vi "Constant Array Size Sha-1.vi"(11 "Message In as Byte Array":u8[](array[numeric])=[97, 0, 0, 0, 0, 0, 0, 0, 0, 0, 0, 0, 0, 0, 0, 0, 0, 0, 0, 0, 0, 0, 0, 0, 0, 0, 0, 0, 0, 0, 0, 0, 0, 0, 0, 0, 0, 0, 0, 0, 0, 0, 0, 0, 0, 0, 0, 0, 0, 0, 0, 0, 0, 0, 0, 0, 0, 0, 0, 0, 0, 0, 0, 0, 0]) -> (3 "Digest":u8[](array[numeric]) format="%x")   [LabVIEW 2014]
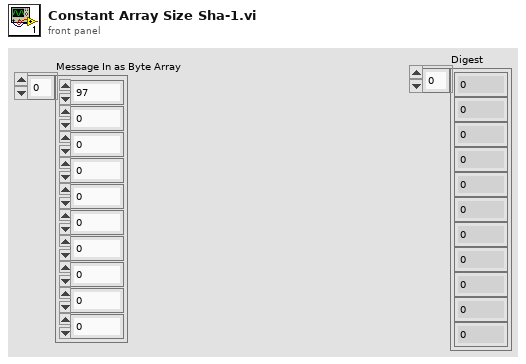
[diagram p1: front panel]
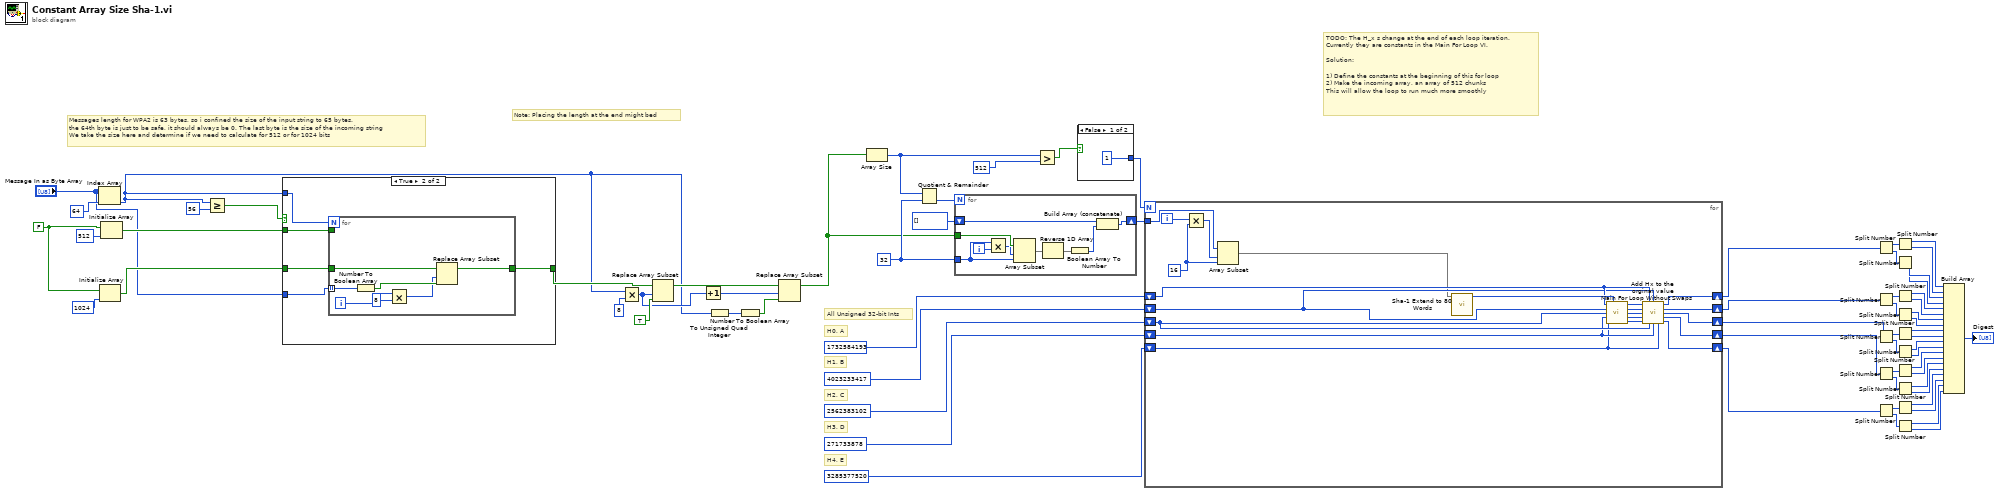
[diagram p0: block diagram]
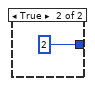
[diagram p2: hidden frame]
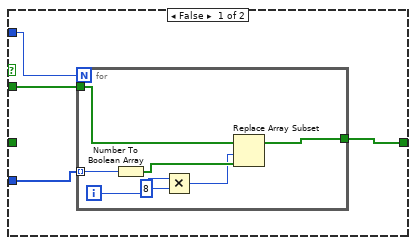
[diagram p3: hidden frame]
diagram:
  w8 = 32 ("y")
  w66 = FALSE
  # "Note: Placing the length at the end might bed"
  # "All Unsigned 32-bit Ints"
  # "H0, A"
  # "H3, D"
  # "H4, E"
  # "H2, C"
  # "H1, B"
  # "TODO: The H_x s change at the end of each loop iteration. \nCurrently they are constants in the Main For Loop VI. \n\nSolution:\n\n1) Define the constants at the beginning of this for loop\n2) Make the incoming array, an array of 512 chunks\nThis will allow the loop to run much more smoothly"
  # "Messages length for WPA2 is 63 bytes, so i confined the size of the input string to 65 bytes. \nthe 64th byte is just to be safe, it should always be 0. The last byte is the size of the incoming string\nWe take the size here and determine if we need to calculate for 512 or for 1024 bits"
  n1 = Index Array(array="Message In as Byte Array", index=64) -> (element=w53:u8)
  n2 = Initialize Array(w66, 1024 ("dimension size")) -> (w62:bool[])
  n3 = Initialize Array(w66, 512 ("dimension size")) -> (w61:bool[])
  n4 = Greater Or Equal?(x=w53, y=u8 56) -> (x >= y?=w63:bool)
  n5 = case shown="True" w63 {
    tunnel: w62 -> [_ w80]
    tunnel: w61 -> [w72 w84]
    tunnel: w53 -> [w70 w81]
    tunnel: "Message In as Byte Array" -> [w71 w83]
    tunnel: [w69 w82] -> w59
    frame False {
      n6 = for {
        N: w70 -> [_]
        tunnel: w72 -> [w78]
        tunnel: w71 -> [w79] mode=indexing
        tunnel: [w73] -> w69
        i -> [w76]
        n7 = Number To Boolean Array(number=w79) -> (Boolean array=w77:bool[])
        n8 = Multiply(x=w76, y=8) -> (x*y=w74:i32)
        n9 = Replace Array Subset(array=w78, new element=w77, index=w74) -> (w73:bool[])
      }
    }
    frame True {
      n10 = for {
        N: w81 -> [_]
        tunnel: w84 -> [_]
        tunnel: w83 -> [w91] mode=indexing
        tunnel: [w86] -> w82
        tunnel: w80 -> [w85]
        i -> [w89]
        n11 = Number To Boolean Array(number=w91) -> (Boolean array=w90:bool[])
        n12 = Multiply(x=w89, y=8) -> (x*y=w87:i32)
        n13 = Replace Array Subset(array=w85, new element=w90, index=w87) -> (w86:bool[])
      }
    }
  }
  n14 = Multiply(x=w53, y=8) -> (x*y=w54:i32)
  n15 = Replace Array Subset(array=w59, new element=TRUE, index=w54) -> (w56:bool[])
  n16 = Increment(x=w54) -> (x+1=w55:i32)
  n17 = To Unsigned Quad Integer(1:w53) -> (0:w52:u64)
  n18 = Number To Boolean Array(number=w52) -> (Boolean array=w51:bool[])
  n19 = Replace Array Subset(array=w56, new element=w51, index=w55) -> (w5:bool[])
  n20 = Array Size(array=w5) -> (size(s)=w3:i32)
  n21 = Quotient & Remainder(x=w3, y=w8) -> (floor(x/y)=w9:i32)  [unwired: 1 out]
  n22 = for {
    N: w9 -> [_]
    tunnel: w5 -> [w100]
    tunnel: w8 -> [w96]
    shift-right: [w94] -> w6
    shift-left: u32[] [] -> [w93]
    i -> [w98]
    n23 = Multiply(x=w96, y=w98) -> (x*y=w97:i32)
    n24 = Array Subset(array=w100, index=w97, length=w96) -> (w99:bool[])
    n25 = Reverse 1D Array(array=w99) -> (reversed array=w95:bool[])
    n26 = Boolean Array To Number(Boolean array=w95) -> (number=w92:u32)
    n27 = Build Array (concatenate)(w93, w92) -> (w94:u32[])
  }
  n28 = Greater?(x=w3, y=512) -> (0:w2:bool)
  n29 = case shown="False" w2 {
    tunnel: [1 2] -> w1
    frame False {
    }
    frame True {
    }
  }
  n30 = for {
    N: w1 -> [_]
    shift-right: [w118] -> w45
    shift-left: u32 1732584193 -> [w112]
    shift-right: [w117] -> w32
    shift-left: u32 4023233417 -> [w111]
    shift-right: [w116] -> w23
    shift-left: u32 2562383102 -> [w110]
    shift-right: [w115] -> w22
    shift-left: u32 271733878 -> [w109]
    shift-right: [w114] -> w19
    shift-left: u32 3285377520 -> [w108]
    tunnel: w6 -> [w104]
    i -> [w107]
    w106 = 16 ("length")
    n31 = Multiply(x=w107, y=w106) -> (x*y=w105:i32)
    n32 = Array Subset(array=w104, index=w105, length=w106) -> (w103:u32[])
    n33 = call "Sha-1 Extend to 80 Words.vi"("16 32-bit Words In"=w103) -> ("80 32 Bit Words Out"=w113:u32[])  [unwired: 10 in]
    n34 = call "Main For Loop Without Swaps.vi"("A"=w112, "80 32-bit Words"=w113, "B"=w111, "C"=w110, "D"=w109, "E"=w108) -> ("A Out"=w123:u32, "B Out"=w122:u32, "C Out"=w121:u32, "D Out"=w120:u32, "E Out"=w119:u32)  [unwired: 5 in]
    n35 = call "Add Hx to the orginal value.vi"("A Out"=w123, "H0 In"=w112, "H1 In"=w111, "B Out"=w122, "C Out"=w121, "D Out"=w120, "E Out"=w119, "H2 In"=w110, "H3 In"=w109, "H4 In"=w108) -> ("H0"=w118:u32, "H1"=w117:u32, "H2"=w116:u32, "H3"=w115:u32, "H4"=w114:u32)  [unwired: 1 in]
  }
  n36 = Split Number(x=w45) -> (hi(x)=w44:u16, lo(x)=w43:u16)
  n37 = Split Number(x=w32) -> (hi(x)=w37:u16, lo(x)=w38:u16)
  n38 = Split Number(x=w23) -> (hi(x)=w30:u16, lo(x)=w31:u16)
  n39 = Split Number(x=w22) -> (hi(x)=w24:u16, lo(x)=w25:u16)
  n40 = Split Number(x=w19) -> (hi(x)=w21:u16, lo(x)=w20:u16)
  n41 = Split Number(x=w44) -> (hi(x)=w42:u8, lo(x)=w41:u8)
  n42 = Split Number(x=w43) -> (hi(x)=w40:u8, lo(x)=w39:u8)
  n43 = Split Number(x=w37) -> (hi(x)=w36:u8, lo(x)=w35:u8)
  n44 = Split Number(x=w38) -> (hi(x)=w34:u8, lo(x)=w33:u8)
  n45 = Split Number(x=w30) -> (hi(x)=w29:u8, lo(x)=w28:u8)
  n46 = Split Number(x=w31) -> (hi(x)=w27:u8, lo(x)=w26:u8)
  n47 = Split Number(x=w24) -> (hi(x)=w18:u8, lo(x)=w17:u8)
  n48 = Split Number(x=w25) -> (hi(x)=w16:u8, lo(x)=w15:u8)
  n49 = Split Number(x=w21) -> (hi(x)=w14:u8, lo(x)=w13:u8)
  n50 = Split Number(x=w20) -> (hi(x)=w12:u8, lo(x)=w11:u8)
  n51 = Build Array(w42, w41, w40, w39, w36, w35, w34, w33, w29, w28, w27, w26, w18, w17, w16, w15, w14, w13, w12, w11) -> (→"Digest":u8[])
